vi "DSF.Memory.Cache.Transfer.Set Buffer.vi"(8 "error in (no error)":errorcluster, 10 "Buffer":refnum<class "DSF.Memory.Buffer.lvclass">, 11 "Transfer Cache in":refnum<class "DSF.Memory.Cache.Transfer.lvclass">) -> (0 "error out":errorcluster, 3 "Transfer Cache out":refnum<class "DSF.Memory.Cache.Transfer.lvclass">)   [LabVIEW 2016, in "DSF.Memory.lvlib" / "DSF.Memory.Cache.Transfer.lvclass"]
uses:
  DSF.Memory.Cache.Transfer.lvclass
  Memory.Buffer/DSF.Memory.Buffer.lvclass
  DSF.Memory.Cache.Transfer.lvclass/DSF.Memory.Cache.Transfer.ctl
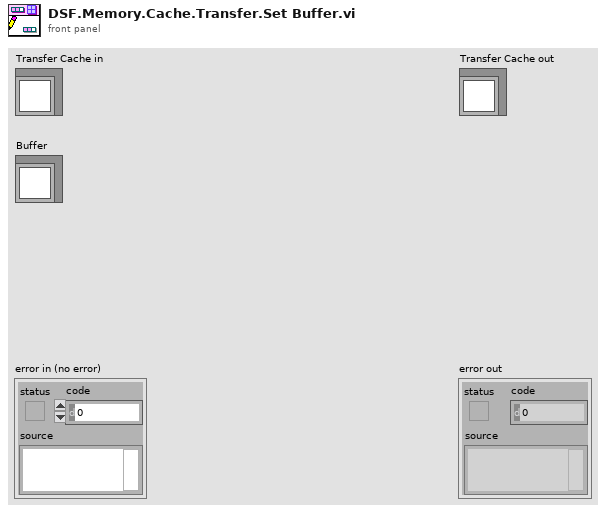
[diagram p1: front panel]
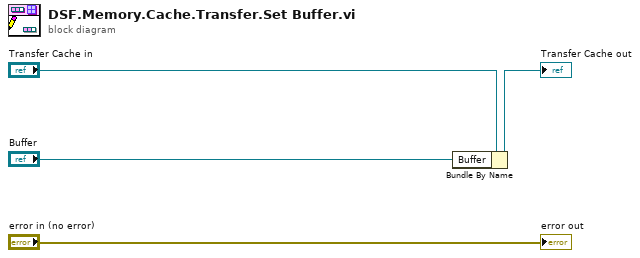
[diagram p0: block diagram]
diagram:
  n1 = Bundle By Name(cluster="Transfer Cache in", "Buffer"="Buffer") -> (→"Transfer Cache out":refnum<class "DSF.Memory.Cache.Transfer.lvclass">)
  "error out" <- "error in (no error)"
